vi "Set All SLSC Switch Properties.vi"(8 "error in (no error)":errorcluster, 10 "SLSC Switch All Properties":T1, 11 "SLSC Switch Custom Device Ref in":T2 format="%.0x") -> (0 "error out":errorcluster, 3 "SLSC Switch Custom Device Ref out":T2 format="%.0x")   [LabVIEW 2017, in "SLSC Switch Scripting.lvlib"]
uses:
  SLSC Switch Scripting.lvlib
  <vilib>/NI Veristand/Custom Device API/Custom Device Item Ref.ctl
  SLSC Switch All Properties.ctl
  <vilib>/NI Veristand/Custom Device API/Custom Device API.lvlib
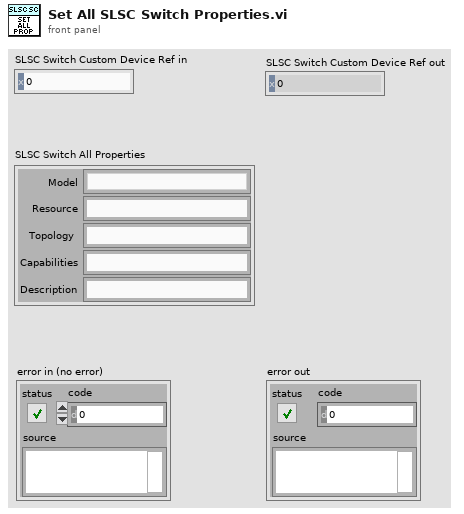
[diagram p1: front panel]
types:
  T1 = typedef "SLSC Switch Scripting.lvlib/SLSC Switch All Properties.ctl" = cluster{"Model":string, "Resource":string, "Topology":string, "Capabilities":string, "Description":string}
  T2 = typedef "Custom Device API.lvlib/Custom Device Item Ref.ctl" = u64
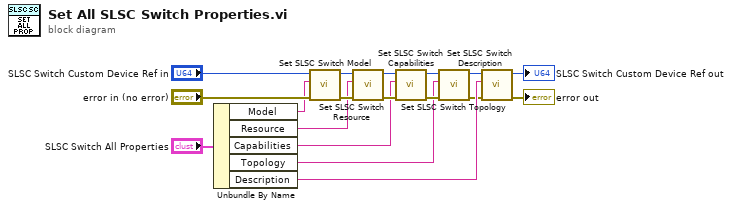
[diagram p0: block diagram]
diagram:
  n1 = Unbundle By Name("SLSC Switch All Properties") -> ("Model"=w12:string, "Resource"=w13:string, "Capabilities"=w5:string, "Topology"=w4:string, "Description"=w9:string)
  n2 = call "Set SLSC Switch Model.vi"("error in (no error)"="error in (no error)", "Model"=w12, "SLSC Switch Custom Device Ref in"="SLSC Switch Custom Device Ref in") -> ("error out"=w18:errorcluster, "SLSC Switch Custom Device Ref out"=w17:T2)  [unwired: 7 in]
  n3 = call "Set SLSC Switch Resource.vi"("error in (no error)"=w18, "Resource"=w13, "SLSC Switch Custom Device Ref in"=w17) -> ("error out"=w8:errorcluster, "SLSC Switch Custom Device Ref out"=w1:T2)  [unwired: 7 in]
  n4 = call "Set SLSC Switch Capabilities.vi"("error in (no error)"=w8, "Capabilities"=w5, "SLSC Switch Custom Device Ref in"=w1) -> ("error out"=w7:errorcluster, "SLSC Switch Custom Device Ref out"=w3:T2)  [unwired: 7 in]
  n5 = call "Set SLSC Switch Topology.vi"("error in (no error)"=w7, "Topology"=w4, "SLSC Switch Custom Device Ref in"=w3) -> ("error out"=w6:errorcluster, "SLSC Switch Custom Device Ref out"=w2:T2)  [unwired: 7 in]
  n6 = call "Set SLSC Switch Description.vi"("error in (no error)"=w6, "Description"=w9, "SLSC Switch Custom Device Ref in"=w2) -> ("error out"=→"error out":errorcluster, "SLSC Switch Custom Device Ref out"=→"SLSC Switch Custom Device Ref out":T2)  [unwired: 7 in]
